vi "PythonFunction.vi"(6 "info":T1, 9 "Python module  name":string, 10 "Python module":string) -> (3 "PythonFunction out":refnum<class "PythonFunction.lvclass">)   [LabVIEW 2014, in "PythonFunction.lvclass"]
uses:
  PythonFunction.lvclass
  DocstringTD.ctl
  PythonFunction.lvclass/PythonFunction.ctl
  Python Functions.lvlib
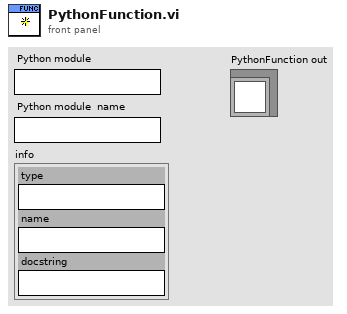
[diagram p1: front panel]
types:
  T1 = typedef "Python Functions.lvlib/DocstringTD.ctl" = cluster{"type":string, "name":string, "docstring":string}
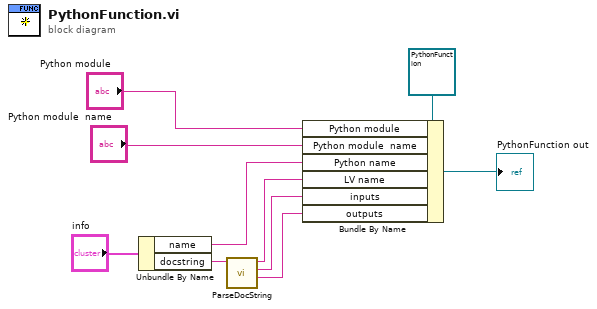
[diagram p0: block diagram]
diagram:
  n1 = Unbundle By Name("info") -> ("name"=w2:string, "docstring"=w8:string)
  n2 = call "ParseDocString.vi"("docstring"=w8) -> ("outputs"=w5:string, "inputs"=w6:string, "function name"=w7:string)  [unwired: 8 in]
  n3 = Bundle By Name(cluster=refnum<class "PythonFunction.lvclass"> refnum ("PythonFunction in"), "Python module"="Python module", "Python module  name"="Python module  name", "Python name"=w2, "LV name"=w7, "inputs"=w6, "outputs"=w5) -> (→"PythonFunction out":refnum<class "PythonFunction.lvclass">)
